vi "通讯全局变量断电保存.vi"() -> ()   [LabVIEW 2016, in "环境动力监测库.lvlib" / "浮标电源管理.lvlib"]
panel:
  in  "控制对象":enum16{"所有辅助设备", "气象电源", "视频电源"}(ring)=enum."视频电源"
  in  "辅助电源控制类型":enum16{"定时控制", "电压控制"}(ring)
  in  "辅助设备电源关闭时间":u16(ring)=12 items=["00H", "01H", "02H", "03H", "04H", "05H", "06H", "07H", "08H", "09H", "10H", "11H", "12H", "13H", "14H", "15H", "16H", "17H", "18H", "19H", "20H", "21H", "22H", "23H"]
  in  "辅助设备电源开启时间":u16(ring)=12 items=["00H", "01H", "02H", "03H", "04H", "05H", "06H", "07H", "08H", "09H", "10H", "11H", "12H", "13H", "14H", "15H", "16H", "17H", "18H", "19H", "20H", "21H", "22H", "23H"]
  in  "开启辅助电源控制":bool
  in  "辅助设备电源开启电压 V":dbl=13.0
  in  "辅助设备电源关闭电压 V":dbl=12.0
  in  "IO模块启用":bool
  in  "串口启用":bool
  in  "VISA Resource":refnum<visa-resource-name>
  in  "报警参数配置":T1={"低压报警阈值 V"=11.0, "低压报警解除阈值 V"=13.0, "高温报警阈值 ℃"=50.0, "高温报警解除阈值 ℃"=40.0, "湿度报警阈值 %"=95.0, "湿度报警解除阈值 %"=90.0}
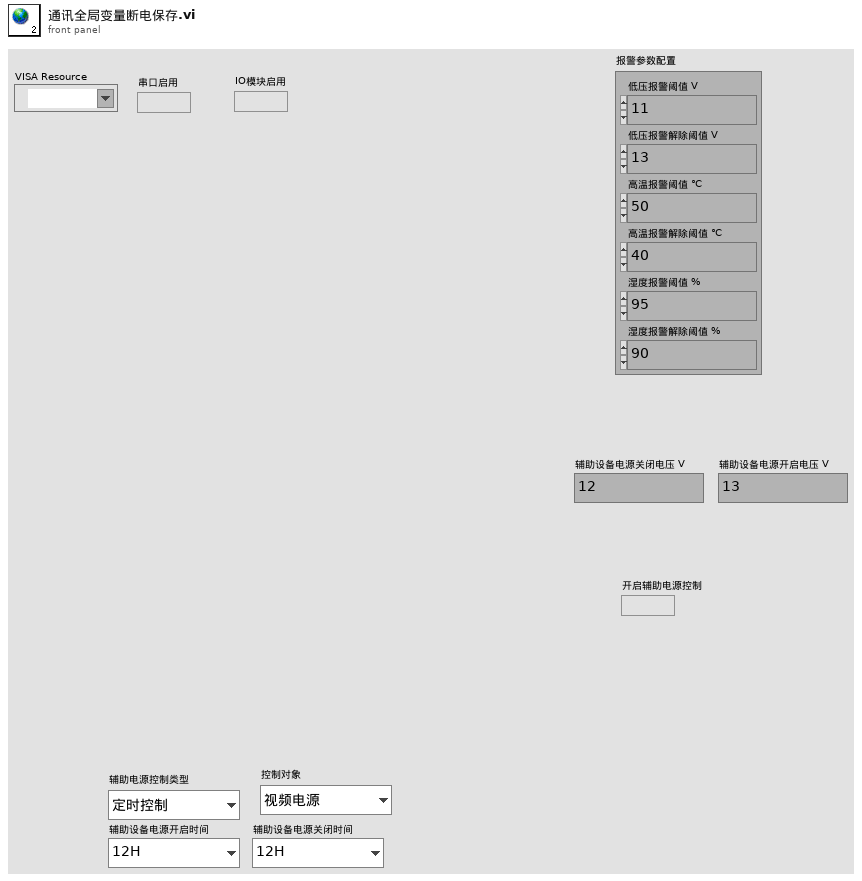
[diagram p1: front panel]
types:
  T1 = cluster{"低压报警阈值 V":dbl, "低压报警解除阈值 V":dbl, "高温报警阈值 ℃":dbl, "高温报警解除阈值 ℃":dbl, "湿度报警阈值 %":dbl, "湿度报警解除阈值 %":dbl}
diagram:
